vi "task1_LED_SWITCH.vi"() -> ()   [LabVIEW 2017]
panel:
  in  "LED7":bool
  in  "LED6":bool
  in  "LED5":bool
  in  "LED4":bool
  in  "LED3":bool
  in  "LED2":bool
  in  "LED1":bool
  in  "LED0":bool
  out "LED7":bool
  out "LED6":bool
  out "LED5":bool
  out "LED4":bool
  out "LED3":bool
  out "LED2":bool
  out "LED1":bool
  out "LED0":bool
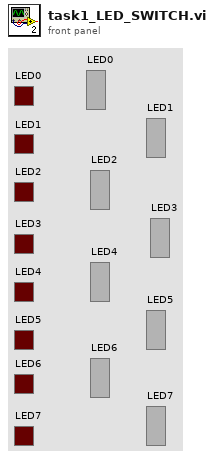
[diagram p1: front panel]
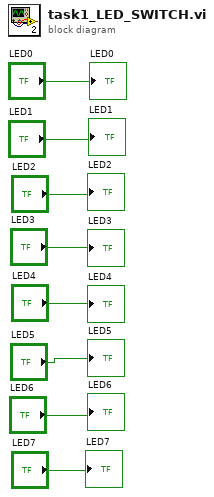
[diagram p0: block diagram]
diagram:
  "LED0" <- "LED0"
  "LED1" <- "LED1"
  "LED2" <- "LED2"
  "LED3" <- "LED3"
  "LED4" <- "LED4"
  "LED5" <- "LED5"
  "LED6" <- "LED6"
  "LED7" <- "LED7"
